vi "Main_xxa.vi"() -> ()   [LabVIEW 2023]
panel:
  out "Answer":u32
  in  "Puzzle":string
  in  "Example":string
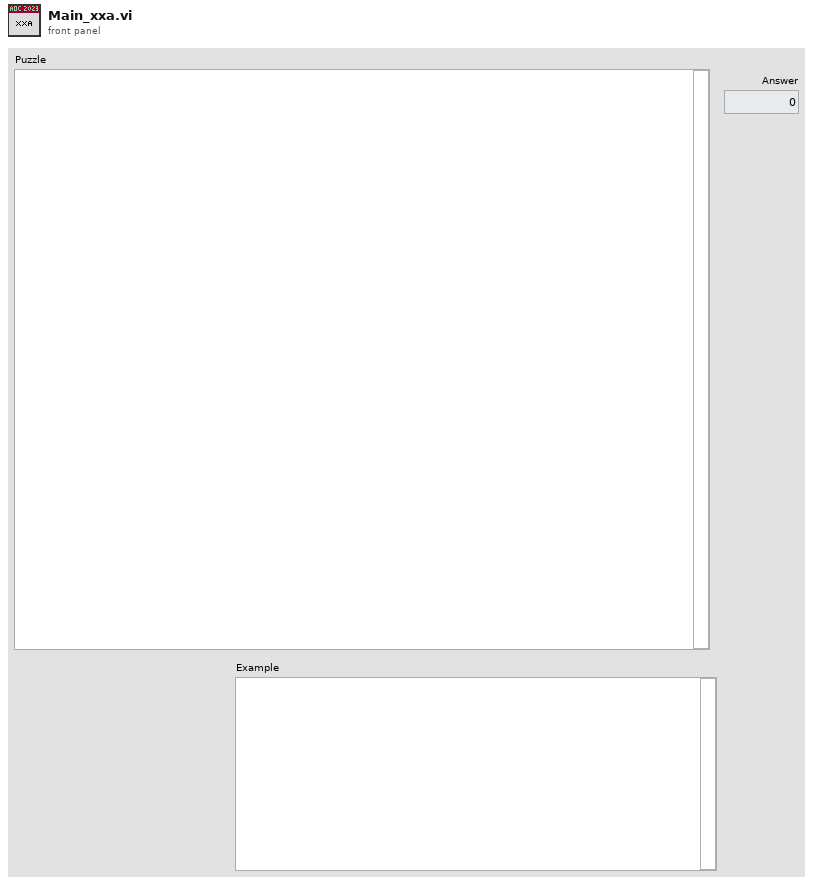
[diagram p1: front panel]
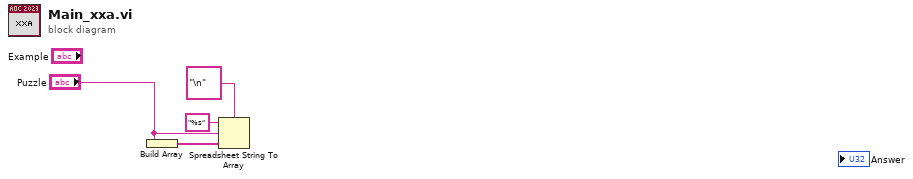
[diagram p0: block diagram]
diagram:
  n1 = Build Array("Puzzle") -> (w4:string[])
  n2 = Spreadsheet String To Array(delimiter (Tab)="\n", format string="%s", spreadsheet string="Puzzle", array type (2D Dbl)=w4) -> ()  [unwired: 1 out]
